vi "Create New.vi"(8 "error in (no error)":errorcluster, 10 "Daemonized":bool=TRUE, 11 "Options":T1) -> (0 "error out":errorcluster, 3 "Execution out":refnum<class "Execution.lvclass">)   [LabVIEW 2020, in "TSnax.lvlib" / "Execution.lvclass"]
uses:
  Execution.lvclass
  Execution.lvclass/Execution.ctl
  Execution Options.ctl
  TSnax.lvlib
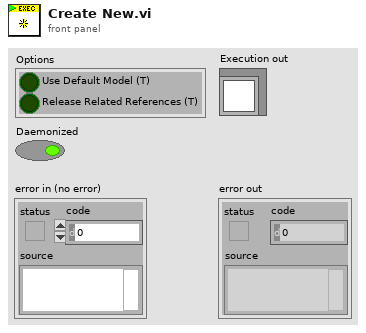
[diagram p1: front panel]
types:
  T1 = typedef "TSnax.lvlib/Execution Options.ctl" = cluster{"Use Default Model (T)":bool, "Release Related References (T)":bool}
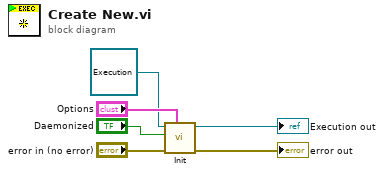
[diagram p0: block diagram]
diagram:
  n1 = call "Init.vi"("Options"="Options", "error in (no error)"="error in (no error)", "Daemonized"="Daemonized", "Execution in"=refnum<class "Execution.lvclass"> refnum) -> ("error out"=→"error out":errorcluster, "Execution out"=→"Execution out":refnum<class "Execution.lvclass">)  [unwired: 6 in]
